vi "Create Hardware Configuration UI.vi"(8 "error in (no error)":errorcluster, 11 "Path":path) -> (0 "error out":errorcluster, 2 "new file?":bool, 3 "name":string)   [LabVIEW 2023]
uses:
  Resources/Type Defs/Stage Configuration.ctl
  Resources/Type Defs/Virtual Camera Configuration.ctl
  Resources/Type Defs/Camera Type.ctl
  Resources/Type Defs/Laser Configuration.ctl
  Resources/Type Defs/Physical Camera Assignment.ctl
  Resources/Type Defs/Microscope Configuration.ctl
  Resources/Type Defs/Microscope Type.ctl
  Resources/Type Defs/DAQ Configuration.ctl
  Resources/Type Defs/Shutter Configuration.ctl
  Resources/Type Defs/Sync Device Type.ctl
  Resources/Type Defs/Hardware Configuration.ctl
  16746906-b5a3-4113-90e7-9719cfb4bdfa.vi
  aeb34b63-e1d6-4ce5-90e9-12bf91c6bf83.vi
  <vilib>/Utility/xml.llb/Read From XML File(string).vi
  <vilib>/JDP Science/JSONtext/JSON text to Variant.vi
  <vilib>/JDP Science/JSONtext/Variant to JSON Text.vi
  <vilib>/Utility/xml.llb/Write to XML File(string).vi
  <vilib>/JDP Science/JSONtext/LVClass Serializer/JSONtext LVClass Serializer.lvclass
panel:
  in  "DAQ Configuration":T1={"Shutters"=[{"IO Line"="\n/line1", "Name"="Cy2", "Wavelength"=473, "Max rate (Hz)"=0.0}, {"IO Line"="Dev1/port1/line1", "Name"="Cy3", "Wavelength"=532, "Max rate (Hz)"=0.0}, {"IO Line"="Dev1/port1/line1", "Name"="Cy5", "Wavelength"=640, "Max rate (Hz)"=0.0}, {"IO Line"="Dev1/port1/line1", "Name"="Cy7", "Wavelength"=721, "Max rate (Hz)"=0.0}], "fluidics trigger line"="Dev1/port1/line1", "camera trigger line"="", "COM Port"="COM3", "Device type"=enum."NI DAQ"}
  in  "Power Meter":T4={"Power Meter Type"=enum."Disabled", "attenuation"=53.2, "instrument handle"=""}
  in  "SaveAs":bool
  in  "Cancel Button":bool
  in  "OK Button":bool
  in  "Microscope":T5={"Serial Port"="COM2", "Microscope Type"=enum."Ti2", "Detection Settings"=[{"Name"="Cy2 (Right)", "Filter Position"=1, "Optical Path"=2}, {"Name"="Cy3 (Right)", "Filter Position"=2, "Optical Path"=2}, {"Name"="Cy5 (Right)", "Filter Position"=3, "Optical Path"=2}, {"Name"="Cy7 (Right)", "Filter Position"=4, "Optical Path"=2}, {"Name"="No Filter (Right)", "Filter Position"=5, "Optical Path"=2}, {"Name"="Lasers to Eyes", "Filter Position"=6, "Optical Path"=1}]}
  in  "Cameras":T7[](array[typedef])=[{"Channel Name"="Cy2", "Serial Number"="000117", "Flip Vertically"=TRUE, "Flip Horizontally"=FALSE, "wavelength"=473, "photonsPerCount"=[]}, {"Channel Name"="Cy3", "Serial Number"="000112", "Flip Vertically"=FALSE, "Flip Horizontally"=FALSE, "wavelength"=532, "photonsPerCount"=[]}, {"Channel Name"="Cy5", "Serial Number"="000113", "Flip Vertically"=FALSE, "Flip Horizontally"=FALSE, "wavelength"=640, "photonsPerCount"=[]}, {"Channel Name"="Cy7", "Serial Number"="000115", "Flip Vertically"=TRUE, "Flip Horizontally"=FALSE, "wavelength"=721, "photonsPerCount"=[]}]
  in  "Lasers":T8[](array[typedef])=[{"Serial Port"="COM6", "Laser Type"=enum."Laser Quantum", "Polarizer Amplitude"=0.0, "Polarizer Theta Zero"=0.0, "Wavelength"=473}, {"Serial Port"="COM4", "Laser Type"=enum."PRM1-Z8", "Polarizer Amplitude"=5791.13, "Polarizer Theta Zero"=-7.65131, "Wavelength"=532}, {"Serial Port"="", "Laser Type"=enum."Coherent HOPS", "Polarizer Amplitude"=0.0, "Polarizer Theta Zero"=0.0, "Wavelength"=640}, {"Serial Port"="", "Laser Type"=enum."Disable", "Polarizer Amplitude"=0.0, "Polarizer Theta Zero"=0.0, "Wavelength"=721}]
  in  "Camera Driver":T9
  in  "Stage":T11={"Serial Port"="COM4", "Forward Step (mm)"=0.45, "Lane Length (mm)"=6.0, "Lane Separation (mm)"=0.45, "Stage Type"=enum."Ti2", "Autofocus Z Planes"=9, "Autofocus Range (um)"=30.0, "Stage Limits"={"Y Min"=-4.5, "Y Max"=3.0, "X Min"=-19.0, "X Max"=33.5}, "Slide (mm)"={"top"=-13.0, "right"=-22.3, "width"=60.0, "height"=25.4}}
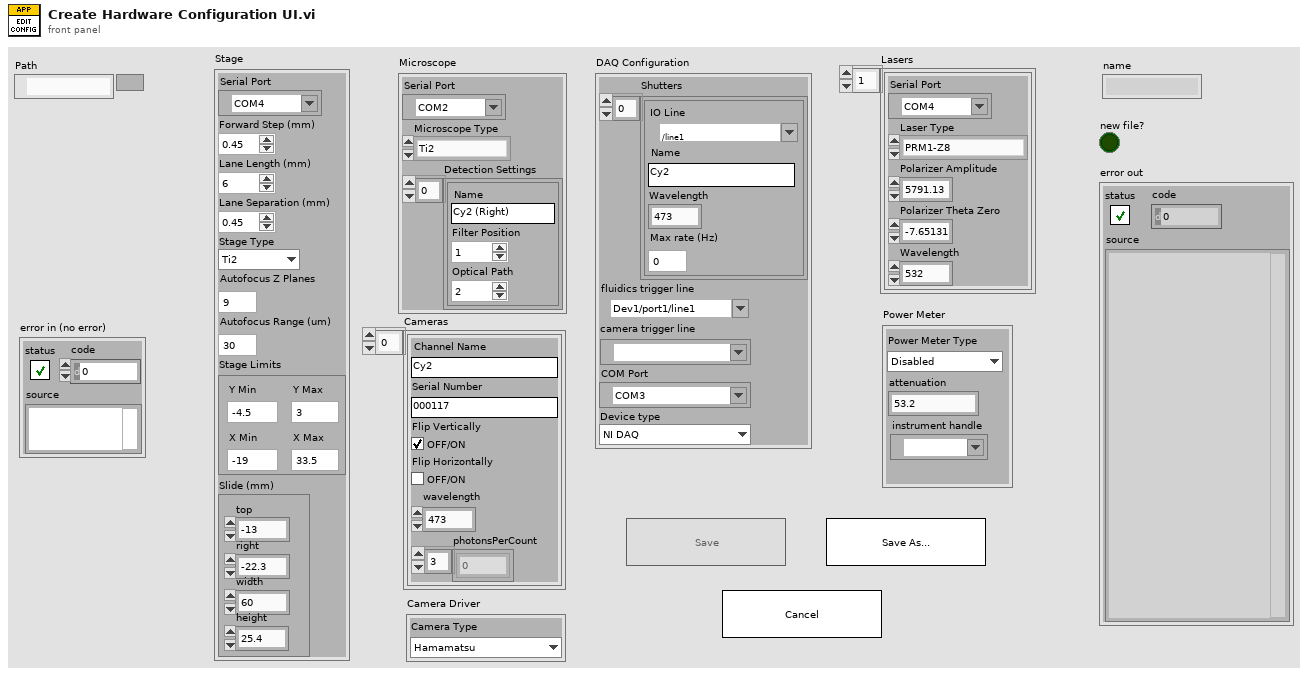
[diagram p1: front panel]
types:
  T1 = typedef "DAQ Configuration.ctl" = cluster{"Shutters":T2[], "fluidics trigger line":tag, "camera trigger line":tag, "COM Port":refnum<visa-resource-name>, "Device type":T3}
  T2 = typedef "Shutter Configuration.ctl" = cluster{"IO Line":tag, "Name":string, "Wavelength":u16, "Max rate (Hz)":dbl}
  T3 = typedef "Sync Device Type.ctl" = enum16{"Disabled", "NI DAQ", "Arduino DAQ"}
  T4 = cluster{"Power Meter Type":enum16{"Disabled", "Thorlabs", "Newport", "Coherent"}, "attenuation":dbl, "instrument handle":refnum<visa-resource-name>}
  T5 = typedef "Microscope Configuration.ctl" = cluster{"Serial Port":refnum<visa-resource-name>, "Microscope Type":T6, "Detection Settings":cluster{"Name":string, "Filter Position":u16, "Optical Path":u16}[]}
  T6 = typedef "Microscope Type.ctl" = enum16{"Disable", "TE2000", "Eclipse Ti", "Ti2"}
  T7 = typedef "Physical Camera Assignment.ctl" = cluster{"Channel Name":string, "Serial Number":string, "Flip Vertically":bool, "Flip Horizontally":bool, "wavelength":i16, "photonsPerCount":dbl[]}
  T8 = typedef "Laser Configuration.ctl" = cluster{"Serial Port":refnum<visa-resource-name>, "Laser Type":enum16{"Disable", "Laser Quantum", "Coherent OBIS", "PRM1-Z8", "Coherent HOPS", "Cobolt"}, "Polarizer Amplitude":dbl, "Polarizer Theta Zero":dbl, "Wavelength":u16}
  T9 = typedef "Virtual Camera Configuration.ctl" = cluster{"Camera Type":T10}
  T10 = typedef "Camera Type.ctl" = enum16{"Hamamatsu", "Andor", "Photometrics"}
  T11 = typedef "Stage Configuration.ctl" = cluster{"Serial Port":refnum<visa-resource-name>, "Forward Step (mm)":dbl, "Lane Length (mm)":dbl, "Lane Separation (mm)":dbl, "Stage Type":enum16{"Disabled", "ESP301", "Ti2", "Ludl", "ASI"}, "Autofocus Z Planes":i32, "Autofocus Range (um)":dbl, "Stage Limits":cluster{"Y Min":dbl, "Y Max":dbl, "X Min":dbl, "X Max":dbl}, "Slide (mm)":cluster{"top":dbl, "right":dbl, "width":dbl, "height":dbl}}
  T12 = enum8{"Enabled", "Disabled", "Disabled and Grayed Out"}
  T13 = typedef "Hardware Configuration.ctl" = cluster{"Stage Configuration":T11, "Microscope Configuration":T5, "Virtual Camera Configuration":T9, "Laser Configuration":T8[], "Installed Cameras":T7[], "Power Meter Configuration":cluster{"Power Meter Type":enum16{"Disabled", "Thorlabs", "Newport", "Coherent"}, "attenuation":dbl, "instrument handle":refnum<visa-resource-name>}, "DAQ Configuration":T1}
  T14 = enum16{"open", "replace", "create", "open or create", "replace or create", "replace or create with confirmation"}
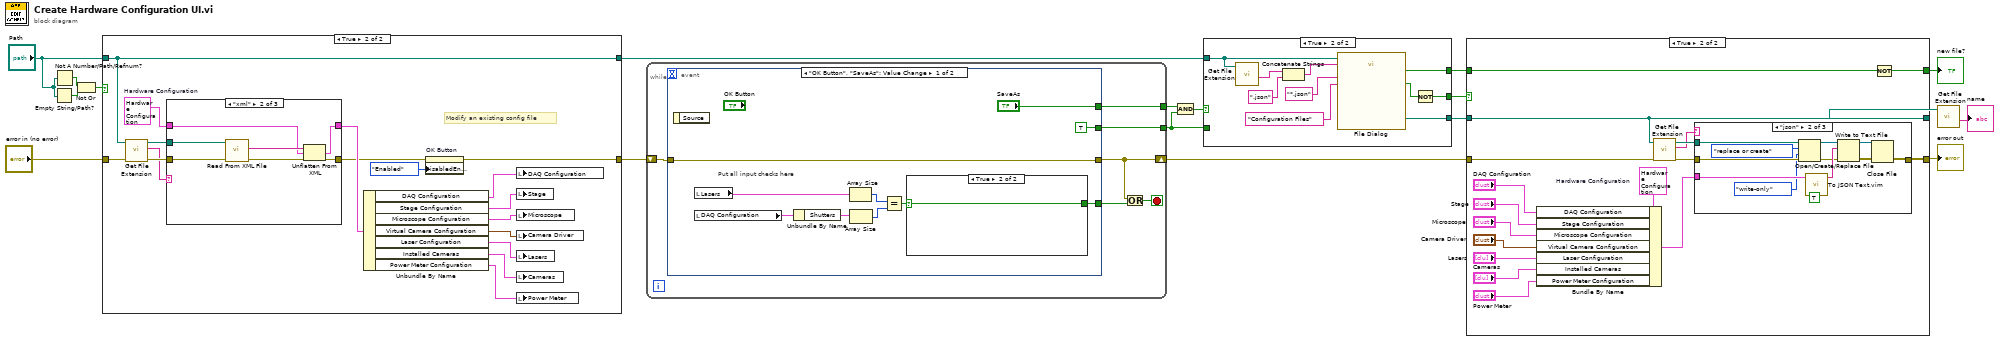
[diagram p0: block diagram]
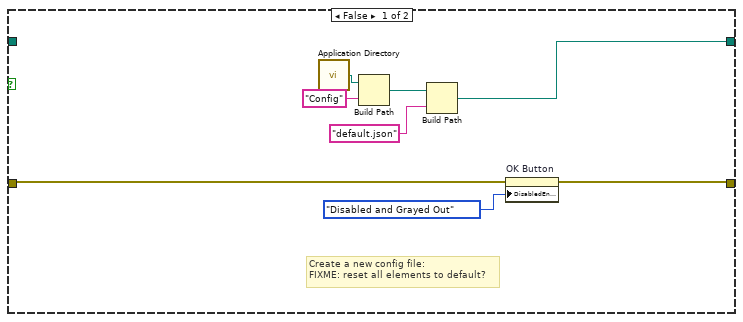
[diagram p2: hidden frame]
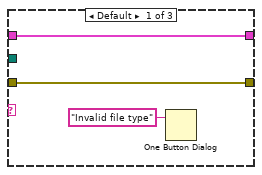
[diagram p3: hidden frame]
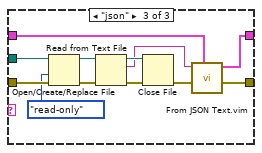
[diagram p4: hidden frame]
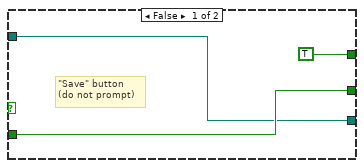
[diagram p5: hidden frame]
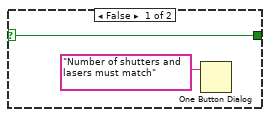
[diagram p6: hidden frame]
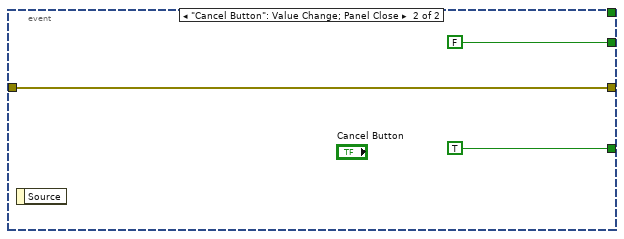
[diagram p7: hidden frame]
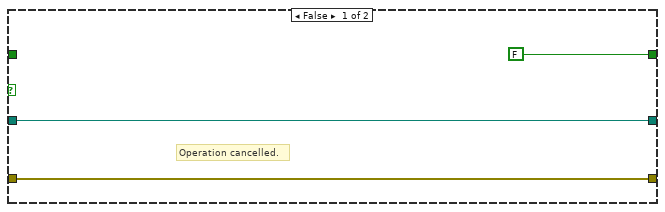
[diagram p8: hidden frame]
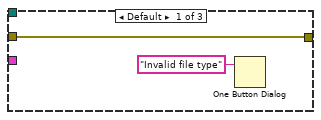
[diagram p9: hidden frame]
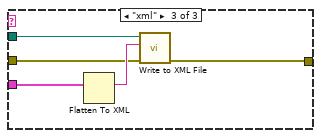
[diagram p10: hidden frame]
diagram:
  n1 = Empty String/Path?(string/path="Path") -> (empty?=w15:bool)
  n2 = Not A Number/Path/Refnum?(number/path/refnum="Path") -> (NaN/Path/Refnum?=w16:bool)
  n3 = Not Or(1:w15, 2:w16) -> (0:w17:bool)
  n4 = case shown="True" w17 {
    tunnel: "Path" -> [_ w30]
    tunnel: "error in (no error)" -> [w21 w32]
    tunnel: [w20 w28] -> w14
    tunnel: [w22 w30] -> w1
    frame False {
      # "Create a new config file:\nFIXME: reset all elements to default?"
      n5 = call <vilib>:"Application Directory.vi"() -> ("Application Directory"=w25:path)
      n6 = Build Path(base path=w25, name or relative path="Config") -> (appended path=w24:path)
      n7 = Build Path(base path=w24, name or relative path="default.json") -> (appended path=w22:path)
      n8 = property on="OK Button" class="Bool"(error in=w21, "DisabledEnum"=T12."Disabled and Grayed Out" ("Disabled")) -> (error out=w20:errorcluster)  [unwired: 1 in, 1 out]
    }
    frame True {
      w43 = T13 {"Stage Configuration"={"Serial Port"="COM3", "Forward Step (mm)"=0.4, "Lane Length (mm)"=6.0, "Lane Separation (mm)"=0.8, "Stage Type"=enum."ESP301", "Autofocus Z Planes"=9, "Autofocus Range (um)"=30.0, "Stage Limits"={"Y Min"=-4.5, "Y Max"=3.0, "X Min"=-19.0, "X Max"=33.5}, "Slide (mm)"={"top"=-22300.0, "right"=-13000.0, "width"=60000.0, "height"=25400.0}}, "Microscope Configuration"={"Serial Port"="COM2", "Microscope Type"=enum."TE2000", "Detection Settings"=[]}, "Virtual Camera Configuration"={"Camera Type"=enum."Hamamatsu"}, "Laser Configuration"=[], "Installed Cameras"=[], "Power Meter Configuration"={"Power Meter Type"=enum."Disabled", "attenuation"=53.2, "instrument handle"="USB0::0x1313::0x8075::P5001392::INSTR"}, "DAQ Configuration"={"Shutters"=[], "fluidics trigger line"="Dev1/port1/line1", "camera trigger line"="", "COM Port"="COM3", "Device type"=enum."NI DAQ"}}  # Hardware Configuration
      # "Modify an existing config file"
      n9 = call <vilib>:"Get File Extension.vi"("error in (no error)"=w32, "file"=w30) -> ("error out"=w33:errorcluster, "lowercase file extension"=w31:string, "dup file"=w34:path)  [unwired: 5 in, 2 out]
      n10 = case shown="\"xml\"" w31 {
        tunnel: w34 -> [_ w53 w60]
        tunnel: w33 -> [w46 w50 w62]
        tunnel: w43 -> [w45 w47 w63]
        tunnel: [w45 w49 w64] -> w42
        tunnel: [w46 w48 w65] -> w29
        frame Default {
          n11 = One Button Dialog(message="Invalid file type") -> ()  [unwired: 1 in, 1 out]
        }
        frame "xml" {
          n12 = call-poly <vilib>:"Read From XML File.vi"("error in (no error)"=w50, "XML File Path"=w53) -> ("error out"=w51:errorcluster, "XML Elements"=w52:string)  [unwired: 7 in, 1 out]
          n13 = Unflatten From XML(xml string=w52, type=w47, error in (no error)=w51) -> (value=w49:T13, error out=w48:errorcluster)
        }
        frame "json" {
          n14 = Open/Create/Replace File(file path (use dialog)=w60, error in=w62, access (0:read/write)=enum16{"read/write", "read-only", "write-only"}."read-only") -> (refnum out=w59:refnum<file>, error out=w61:errorcluster)  [unwired: 3 in, 1 out]
          n15 = Read from Text File(file (use dialog)=w59, error in=w61) -> (refnum out=w57:refnum<file>, text=w56:string, error out=w58:errorcluster)  [unwired: 2 in, 1 out]
          n16 = Close File(refnum=w57, error in=w58) -> (error out=w55:errorcluster)  [unwired: 1 out]
          n17 = call "From JSON Text.vim"("Data Type and Default Value"=w63, "error in (no error)"=w55, "JSON"=w56) -> ("error out"=w65:errorcluster, "Data out"=w64:T13)  [unwired: 7 in]
        }
      }
      n18 = Unbundle By Name(w42) -> ("DAQ Configuration"=w35:T1, "Stage Configuration"=w41:T11, "Microscope Configuration"=w40:T5, "Virtual Camera Configuration"=w39:T9, "Laser Configuration"=w38:T8[], "Installed Cameras"=w37:T7[], "Power Meter Configuration"=w36:T4)
      n19 = property on="OK Button" class="Bool"(error in=w29, "DisabledEnum"=T12."Enabled" ("Disabled")) -> (error out=w28:errorcluster)  [unwired: 1 in, 1 out]
      n20 = local write "DAQ Configuration"(w35) -> ()
      n21 = local write "Stage"(w41) -> ()
      n22 = local write "Microscope"(w40) -> ()
      n23 = local write "Camera Driver"(w39) -> ()
      n24 = local write "Lasers"(w38) -> ()
      n25 = local write "Cameras"(w37) -> ()
      n26 = local write "Power Meter"(w36) -> ()
    }
  }
  n27 = while {
    tunnel: [w70] -> w9
    shift-right: [w66] -> w13
    shift-left: w14 -> [w71]
    tunnel: [w69] -> w11
    stop <- w68 stop-if-true
    n28 = event shown="[0] \"OK Button\", \"SaveAs\": Value Change" {
      selector: _ -> [_ _]
      dyn-events: _ -> [_ _]
      timeout: _ -> [_ _]
      tunnel: w71 -> [w81 w86]
      tunnel: [w81 w86] -> w66
      tunnel: [TRUE FALSE] -> w70
      tunnel: [w75 TRUE] -> w67
      tunnel: ["SaveAs" _] -> w69
      event "OK Button", "SaveAs": Value Change {
        # "Put all input checks here"
        n29 = event-data() -> ()  [unwired: 1 in, 1 out]
        n30 = local read "Lasers"() -> (w79:T8[])
        n31 = local read "DAQ Configuration"() -> (w72:T1)
        n32 = Unbundle By Name(w72) -> ("Shutters"=w73:T2[])
        n33 = Array Size(array=w79) -> (size(s)=w78:i32)
        n34 = Array Size(array=w73) -> (size(s)=w77:i32)
        n35 = Equal?(x=w78, y=w77) -> (x = y?=w76:bool)
        n36 = case shown="True" w76 {
          selector: w76 -> [w83 w84]
          tunnel: [w83 w84] -> w75
          frame False {
            n37 = One Button Dialog(message="Number of shutters and lasers must match") -> ()  [unwired: 1 in, 1 out]
          }
          frame True {
          }
        }
      }
      event "Cancel Button": Value Change; Panel Close {
        n38 = event-data() -> ()  [unwired: 1 in, 1 out]
      }
    }
    n39 = Or(x=w66, y=w67) -> (x .or. y?=w68:bool)
  }
  n40 = And(x=w11, y=w9) -> (x .and. y?=w10:bool)
  n41 = case shown="True" w10 {
    tunnel: [w90 w96] -> w7
    tunnel: w9 -> [w90 _]
    tunnel: w1 -> [w89 w97]
    tunnel: [w89 w100] -> w8
    tunnel: [TRUE ("exists") w98] -> w6
    frame False {
      # "\"Save\" button\n(do not prompt)"
    }
    frame True {
      n42 = call <vilib>:"Get File Extension.vi"("file"=w97) -> ("filename without extension"=w91:string)  [unwired: 6 in, 4 out]
      n43 = Concatenate Strings(w91, ".json" ("string")) -> (w94:string)
      n44 = call "File Dialog"("start path"=w97, "default name"=w94, "pattern (all files)"="*.json", "pattern label"="Configuration Files") -> ("selected path"=w100:path, "exists"=w98:bool, "cancelled"=w95:bool)  [unwired: 8 in, 1 out]
      n45 = Not(x=w95) -> (.not. x?=w96:bool)
    }
  }
  n46 = case shown="True" w7 {
    tunnel: w13 -> [w103 w110]
    tunnel: w8 -> [w102 w108]
    tunnel: [w103 w111] -> w12
    tunnel: [w102 w108] -> w4
    tunnel: w6 -> [_ w104]
    tunnel: [FALSE ("exists") w105] -> w5
    frame False {
      # "Operation cancelled."
    }
    frame True {
      w113 = T13 {"Stage Configuration"={"Serial Port"="COM3", "Forward Step (mm)"=0.4, "Lane Length (mm)"=6.0, "Lane Separation (mm)"=0.8, "Stage Type"=enum."ESP301", "Autofocus Z Planes"=9, "Autofocus Range (um)"=30.0, "Stage Limits"={"Y Min"=-4.5, "Y Max"=3.0, "X Min"=-19.0, "X Max"=33.5}, "Slide (mm)"={"top"=-22300.0, "right"=-13000.0, "width"=60000.0, "height"=25400.0}}, "Microscope Configuration"={"Serial Port"="COM2", "Microscope Type"=enum."TE2000", "Detection Settings"=[]}, "Virtual Camera Configuration"={"Camera Type"=enum."Hamamatsu"}, "Laser Configuration"=[], "Installed Cameras"=[], "Power Meter Configuration"={"Power Meter Type"=enum."Disabled", "attenuation"=53.2, "instrument handle"="USB0::0x1313::0x8075::P5001392::INSTR"}, "DAQ Configuration"={"Shutters"=[], "fluidics trigger line"="Dev1/port1/line1", "camera trigger line"="", "COM Port"="COM3", "Device type"=enum."NI DAQ"}}  # Hardware Configuration
      n47 = Bundle By Name(cluster=w113, "DAQ Configuration"="DAQ Configuration", "Stage Configuration"="Stage", "Microscope Configuration"="Microscope", "Virtual Camera Configuration"="Camera Driver", "Laser Configuration"="Lasers", "Installed Cameras"="Cameras", "Power Meter Configuration"="Power Meter") -> (w112:T13)
      n48 = call <vilib>:"Get File Extension.vi"("error in (no error)"=w110, "file"=w108) -> ("error out"=w109:errorcluster, "lowercase file extension"=w106:string, "dup file"=w107:path)  [unwired: 5 in, 2 out]
      n49 = case shown="\"json\"" w106 {
        tunnel: w112 -> [_ w133 w137]
        tunnel: [w122 w129 w135] -> w111
        tunnel: w109 -> [w122 w127 w136]
        tunnel: w107 -> [_ w126 w139]
        frame Default {
          n50 = One Button Dialog(message="Invalid file type") -> ()  [unwired: 1 in, 1 out]
        }
        frame "json" {
          n51 = Open/Create/Replace File(file path (use dialog)=w126, error in=w127, operation (0:open)=T14."replace or create", access (0:read/write)=enum16{"read/write", "read-only", "write-only"}."write-only") -> (refnum out=w128:refnum<file>, error out=w125:errorcluster)  [unwired: 2 in, 1 out]
          n52 = call "To JSON Text.vim"("Pretty Print?"=TRUE, "Anything"=w133) -> ("<JSON>"=w132:string)  [unwired: 8 in, 1 out]
          n53 = Write to Text File(file (use dialog)=w128, text=w132, error in=w125) -> (refnum out=w130:refnum<file>, error out=w131:errorcluster)  [unwired: 1 in, 1 out]
          n54 = Close File(refnum=w130, error in=w131) -> (error out=w129:errorcluster)  [unwired: 1 out]
        }
        frame "xml" {
          n55 = Flatten To XML(6:w137) -> (2:w138:string)
          n56 = call-poly <vilib>:"Write to XML File.vi"("error in (no error)"=w136, "XML Input"=w138, "XML File Path"=w139) -> ("error out"=w135:errorcluster)  [unwired: 6 in, 2 out]
        }
      }
      n57 = Not(x=w104) -> (.not. x?=w105:bool)
    }
  }
  "error out" <- w12
  "new file?" <- w5
  n58 = call <vilib>:"Get File Extension.vi"("file"=w4) -> ("filename without extension"=→"name":string)  [unwired: 6 in, 4 out]
